vi "testVI.vi"() -> ()   [LabVIEW 2016]
uses:
  Initialize (Remote NVMEM Area).vi
  SLSC Remote.lvclass
  SLSC Interface Class/SLSC Interface.lvclass
panel:
  out "NVMEMArea.Size":u32
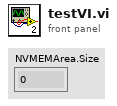
[diagram p1: front panel]
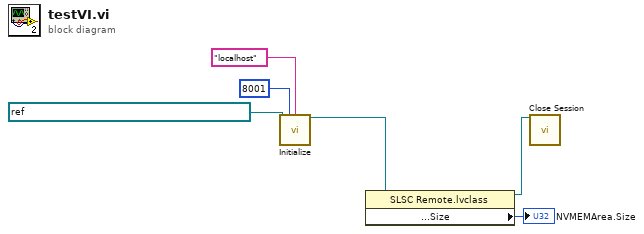
[diagram p0: block diagram]
diagram:
  n1 = call-poly "Initialize.vi"("NVMEM areas"=refnum<k21> "SLSC-12001-030FF53E-Mod2/capabilities", "Port"=u16 8001, "Hostname/IP"="localhost") -> ("SLSC Remote out"=w1:refnum<class "SLSC Remote.lvclass">)  [unwired: 11 in, 1 out]
  n2 = property class="SLSC Remote.lvclass"(reference=w1) -> (reference out=w3:refnum<class "SLSC Remote.lvclass">, "session property node:NVMEM Area:NVMEMArea.Size"=→"NVMEMArea.Size":u32)  [unwired: 1 in, 1 out]
  n3 = call-dynamic "Close Session.vi"("SLSC Remote in"=w3) -> ()  [unwired: 14 in, 1 out]
